vi "1D String Array To String.vi"(11 "Array[]":string[](array[string])) -> (3 "String":string)   [LabVIEW 2023, in "SLL Environment Variable.lvlib"]
doc: "Convert 1D array to string."
uses:
  SLL Environment Variable.lvlib
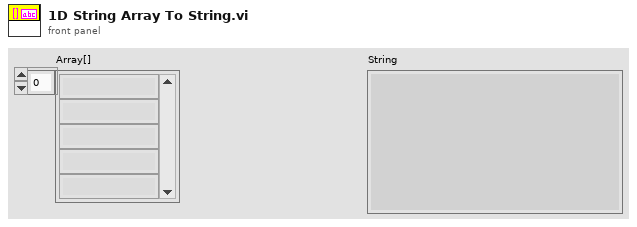
[diagram p1: front panel]
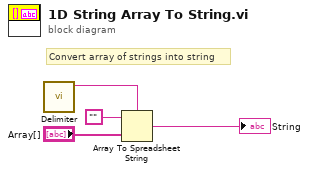
[diagram p0: block diagram]
diagram:
  # "Convert array of strings into string"
  n1 = call "Delimiter.vi"() -> ("Delimiter"=w1:string)  [unwired: 11 in]
  n2 = Array To Spreadsheet String(delimiter (Tab)=w1, array="Array[]", 3:"") -> (spreadsheet string=→"String":string)
